vi "IO檔 Enum name 轉換_20200804.vi"() -> ()   [LabVIEW 2019]
uses:
  <vilib>/Utility/file.llb/Read Delimited Spreadsheet (string).vi
panel:
  out "subarray 2":string[](array[string])
  out "subarray":string[](array[string])
  in  "file path (dialog if empty)":path=path "D:/cubtestcsv.csv"
  out "all rows":string[][](array[string])
  out "Array 2":string[](array[string])
  out "Array":string[](array[string])
  in  "Enum":T1(ring)
  in  "Ring":T2 items=["S1-檢平確認氣缸 (設定值)", "$S1_PreventionChk 1", "S1 電路板檢平On次數(設定值)", "$S1_PreventionChk 2", "S1 電池檢平On次數(設定值)", "$S1_PreventionChk 3", "S1 盒蓋檢平On次數(設定值)", "$S1_PreventionChk 4", "S2電流量測 探針使用次數(設定值)", "$S2_PreventionChk 1", "S2-電流量測氣缸 (設定值)", "$S2_PreventionChk 2", "S3程式燒入 探針使用次數(設定值)", "$S3_PreventionChk 1", "S3-程式燒入氣缸 (設定值)", "$S3_PreventionChk 2", "S4電壓量測探針使用次數(設定值)", "$S4_PreventionChk 1", "S4電源3V探針使用次數(設定值)", "$S4_PreventionChk 2", "S4 隔離箱上蓋氣缸 (設定值)", "$S4_PreventionChk 3", "S4 隔離箱下蓋氣缸 (設定值)", "$S4_PreventionChk 4", "S4 電池電壓量測固定氣缸 (設定值)", "$S4_PreventionChk 5", "S4 電池電壓量測氣缸 (設定值)", "$S4_PreventionChk 6", "S4 電路板檢測氣缸(設定值)", "$S4_PreventionChk 7", "S5 電路板取料升降氣缸 (設定值)", "$S5_PreventionChk 1", "S5 電路板取料橫移氣缸 (設定值)", "$S5_PreventionChk 2", "S5 真空 吸取(設定值)", "$S5_PreventionChk 3", "S5 真空 解除(設定值)", "$S5_PreventionChk 4", "S7 焊接料件固定氣缸 (設定值)", "$S7_PreventionChk 1", "S7 焊接機清錫馬達 (設定值)", "$S7_PreventionChk 2", "S10 料件翻轉區升降氣缸 (設定值)", "$S10_PreventionChk 1", "S10 料件翻轉區伸出氣缸 (設定值)", "$S10_PreventionChk 2", "S10 料件翻轉區旋轉氣缸 (設定值)", "$S10_PreventionChk 3", "S10 料件翻轉區夾取氣缸 (設定值)", "$S10_PreventionChk 4", "S10 料件橫移氣缸 (設定值)", "$S10_PreventionChk 5", "S10 料件吸取升降氣缸 (設定值)", "$S10_PreventionChk 6", "S10 料件放料升降氣缸 (設定值)", "$S10_PreventionChk 7", "S10 真空 吸取(設定值)", "$S10_PreventionChk 8", "S10 真空 解除(設定值)", "$S10_PreventionChk 9", "S11 雷射測高檢知氣缸 (設定值)", "$S11_PreventionChk 1", "S12 熱熔升降氣缸 (設定值)", "$S12_PreventionChk 1", "S12 預熱升降氣缸 (設定值)", "$S12_PreventionChk 2", "S12 離子槍風速調控 (設定值)", "$S12_PreventionChk 3", "S13 真空 吸取 (設定值)", "$S13_PreventionChk 1", "S13 真空 解除(設定值)", "$S13_PreventionChk 2", "S13 NG蓋取料夾爪 (設定值)", "$S13_PreventionChk 3", "S13 NG蓋取料升降 (設定值)", "$S13_PreventionChk 4", "S13 NG電池取料升降 (設定值)", "$S13_PreventionChk 5", "S13 NG電路板取料升降 (設定值)", "$S13_PreventionChk 6", "S13 NG橫移氣缸 (設定值)", "$S13_PreventionChk 7", "S13 NG橫移氣缸(設定值)", "$S13_PreventionChk 8", "S7 焊接啟動次數(設定值)", "$S7_PreventionChk 1", "S12 熱熔次數(設定值)", "$S12_PreventionChk 1", "S11 雷射檢測次數(設定值)", "$S11_PreventionChk 1"]
  in  "DIO":cluster{"DI=1":i32, "Name":string[]}[](array[cluster])
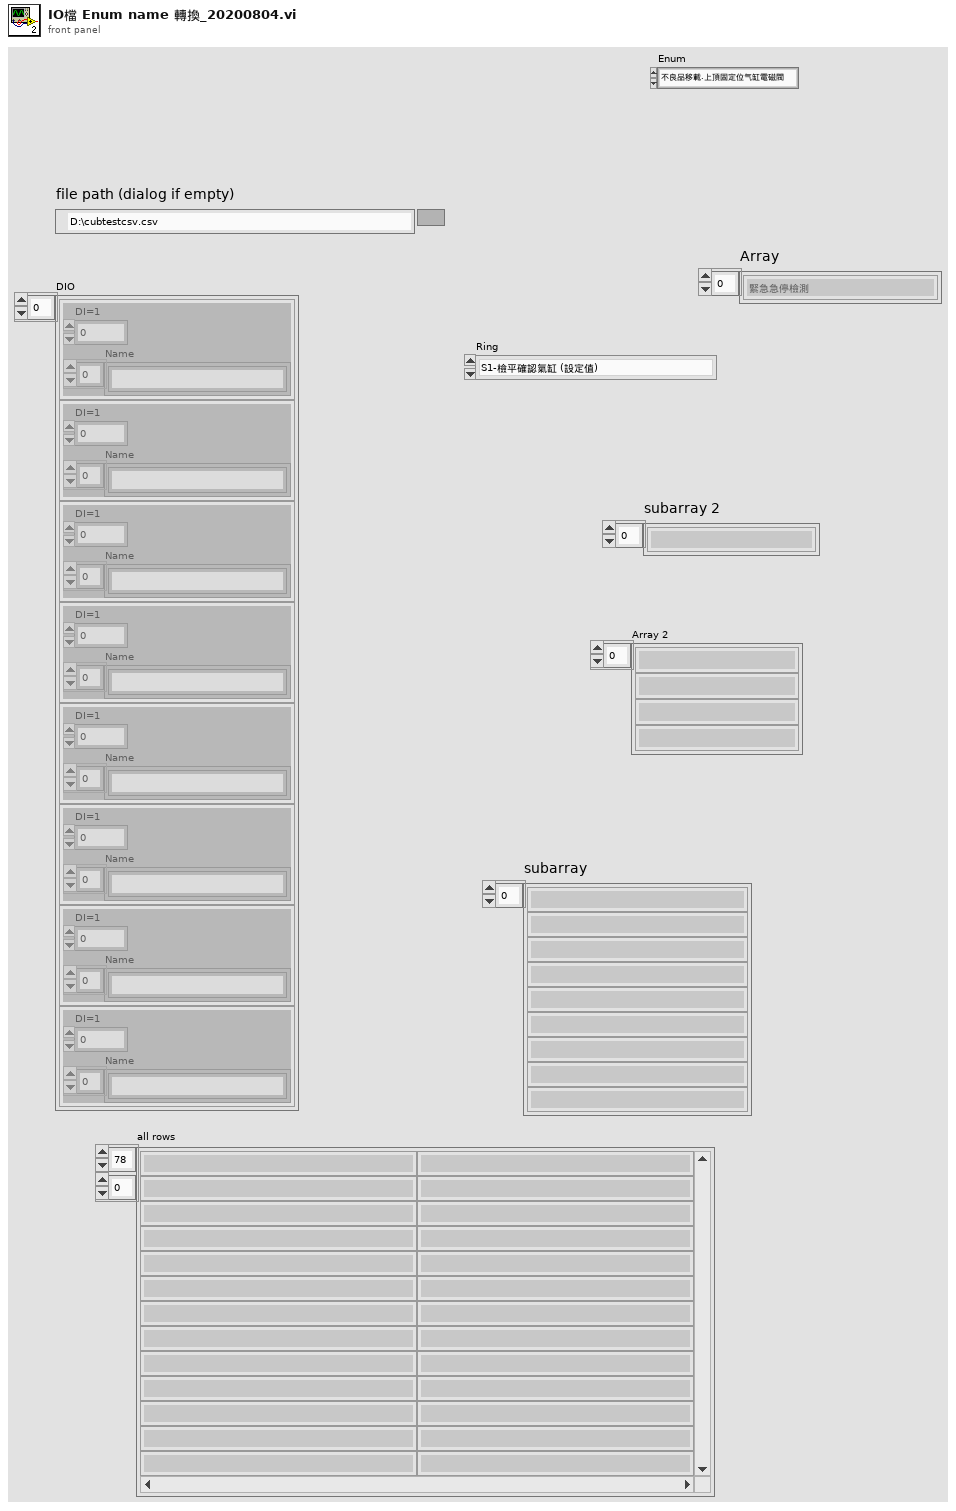
[diagram p1: front panel]
types:
  T1 = enum16{"不良品移載.上頂固定位气缸電磁閥", "不良品移載出料.下壓1氣缸電磁閥", "不良品移載進料.下壓2氣缸電磁閥", "不良品移載.推出料氣缸電磁閥", "不良品移載.推進料氣缸電磁閥"}
  T2 = typedef "預防保養02.ctl" = u16
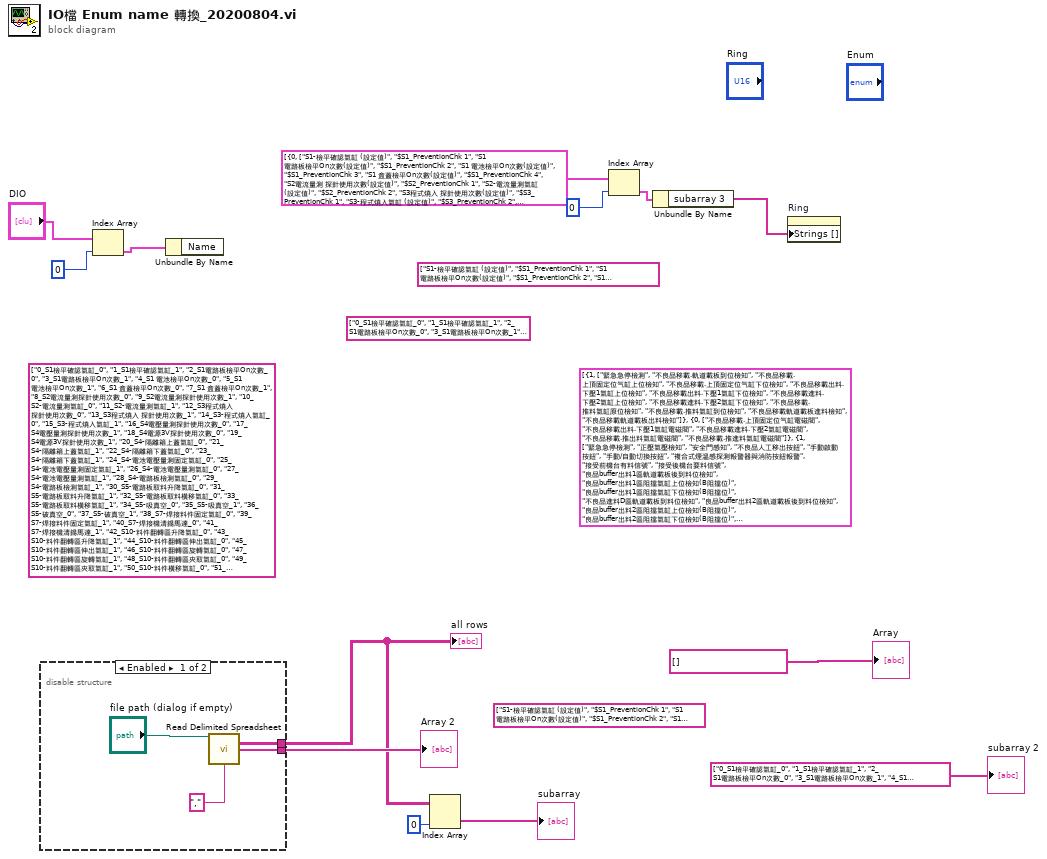
[diagram p0: block diagram]
diagram:
  (unwired) string[] ["S1-檢平確認氣缸 (設定值)", "$S1_PreventionChk 1", "S1 電路板檢平On次數(設定值)", "$S1_PreventionChk 2", "S1 電池檢平On次數(設定值)", "$S1_PreventionChk 3", "S1 盒蓋檢平On次數(設定值)", "$S1_PreventionChk 4", "S2電流量測 探針使用次數(設定值)", "$S2_PreventionChk 1", "S2-電流量測氣缸 (設定值)", "$S2_PreventionChk 2", "S3程式燒入 探針使用次數(設定值)", "$S3_PreventionChk 1", "S3-程式燒入氣缸 (設定值)", "$S3_PreventionChk 2", "S4電壓量測探針使用次數(設定值)", "$S4_PreventionChk 1", "S4電源3V探針使用次數(設定值)", "$S4_PreventionChk 2", "S4 隔離箱上蓋氣缸 (設定值)", "$S4_PreventionChk 3", "S4 隔離箱下蓋氣缸 (設定值)", "$S4_PreventionChk 4", "S4 電池電壓量測固定氣缸 (設定值)", "$S4_PreventionChk 5", "S4 電池電壓量測氣缸 (設定值)", "$S4_PreventionChk 6", "S4 電路板檢測氣缸(設定值)", "$S4_PreventionChk 7", "S5 電路板取料升降氣缸 (設定值)", "$S5_PreventionChk 1", "S5 電路板取料橫移氣缸 (設定值)", "$S5_PreventionChk 2", "S5 真空 吸取(設定值)", "$S5_PreventionChk 3", "S5 真空 解除(設定值)", "$S5_PreventionChk 4", "S7 焊接料件固定氣缸 (設定值)", "$S7_PreventionChk 1", "S7 焊接機清錫馬達 (設定值)", "$S7_PreventionChk 2", "S10 料件翻轉區升降氣缸 (設定值)", "$S10_PreventionChk 1", "S10 料件翻轉區伸出氣缸 (設定值)", "$S10_PreventionChk 2", "S10 料件翻轉區旋轉氣缸 (設定值)", "$S10_PreventionChk 3", "S10 料件翻轉區夾取氣缸 (設定值)", "$S10_PreventionChk 4", "S10 料件橫移氣缸 (設定值)", "$S10_PreventionChk 5", "S10 料件吸取升降氣缸 (設定值)", "$S10_PreventionChk 6", "S10 料件放料升降氣缸 (設定值)", "$S10_PreventionChk 7", "S10 真空 吸取(設定值)", "$S10_PreventionChk 8", "S10 真空 解除(設定值)", "$S10_PreventionChk 9", "S11 雷射測高檢知氣缸 (設定值)", "$S11_PreventionChk 1", "S12 熱熔升降氣缸 (設定值)", "$S12_PreventionChk 1", "S12 預熱升降氣缸 (設定值)", "$S12_PreventionChk 2", "S12 離子槍風速調控 (設定值)", "$S12_PreventionChk 3", "S13 真空 吸取 (設定值)", "$S13_PreventionChk 1", "S13 真空 解除(設定值)", "$S13_PreventionChk 2", "S13 NG蓋取料夾爪 (設定值)", "$S13_PreventionChk 3", "S13 NG蓋取料升降 (設定值)", "$S13_PreventionChk 4", "S13 NG電池取料升降 (設定值)", "$S13_PreventionChk 5", "S13 NG電路板取料升降 (設定值)", "$S13_PreventionChk 6", "S13 NG橫移氣缸 (設定值)", "$S13_PreventionChk 7", "S13 NG橫移氣缸(設定值)", "$S13_PreventionChk 8", "S7 焊接啟動次數(設定值)", "$S7_PreventionChk 1", "S12 熱熔次數(設定值)", "$S12_PreventionChk 4", "S11 雷射檢測次數(設定值)", "$S11_PreventionChk 1"] ("subarray 3")
  (unwired) string[] ["S1-檢平確認氣缸 (設定值)", "$S1_PreventionChk 1", "S1 電路板檢平On次數(設定值)", "$S1_PreventionChk 2", "S1 電池檢平On次數(設定值)", "$S1_PreventionChk 3", "S1 盒蓋檢平On次數(設定值)", "$S1_PreventionChk 4", "S2電流量測 探針使用次數(設定值)", "$S2_PreventionChk 1", "S2-電流量測氣缸 (設定值)", "$S2_PreventionChk 2", "S3程式燒入 探針使用次數(設定值)", "$S3_PreventionChk 1", "S3-程式燒入氣缸 (設定值)", "$S3_PreventionChk 2", "S4電壓量測探針使用次數(設定值)", "$S4_PreventionChk 1", "S4電源3V探針使用次數(設定值)", "$S4_PreventionChk 2", "S4 隔離箱上蓋氣缸 (設定值)", "$S4_PreventionChk 3", "S4 隔離箱下蓋氣缸 (設定值)", "$S4_PreventionChk 4", "S4 電池電壓量測固定氣缸 (設定值)", "$S4_PreventionChk 5", "S4 電池電壓量測氣缸 (設定值)", "$S4_PreventionChk 6", "S4 電路板檢測氣缸(設定值)", "$S4_PreventionChk 7", "S5 電路板取料升降氣缸 (設定值)", "$S5_PreventionChk 1", "S5 電路板取料橫移氣缸 (設定值)", "$S5_PreventionChk 2", "S5 真空 吸取(設定值)", "$S5_PreventionChk 3", "S5 真空 解除(設定值)", "$S5_PreventionChk 4", "S7 焊接料件固定氣缸 (設定值)", "$S7_PreventionChk 1", "S7 焊接機清錫馬達 (設定值)", "$S7_PreventionChk 2", "S10 料件翻轉區升降氣缸 (設定值)", "$S10_PreventionChk 1", "S10 料件翻轉區伸出氣缸 (設定值)", "$S10_PreventionChk 2", "S10 料件翻轉區旋轉氣缸 (設定值)", "$S10_PreventionChk 3", "S10 料件翻轉區夾取氣缸 (設定值)", "$S10_PreventionChk 4", "S10 料件橫移氣缸 (設定值)", "$S10_PreventionChk 5", "S10 料件吸取升降氣缸 (設定值)", "$S10_PreventionChk 6", "S10 料件放料升降氣缸 (設定值)", "$S10_PreventionChk 7", "S10 真空 吸取(設定值)", "$S10_PreventionChk 8", "S10 真空 解除(設定值)", "$S10_PreventionChk 9", "S11 雷射測高檢知氣缸 (設定值)", "$S11_PreventionChk 1", "S12 熱熔升降氣缸 (設定值)", "$S12_PreventionChk 1", "S12 預熱升降氣缸 (設定值)", "$S12_PreventionChk 2", "S12 離子槍風速調控 (設定值)", "$S12_PreventionChk 3", "S13 真空 吸取 (設定值)", "$S13_PreventionChk 1", "S13 真空 解除(設定值)", "$S13_PreventionChk 2", "S13 NG蓋取料夾爪 (設定值)", "$S13_PreventionChk 3", "S13 NG蓋取料升降 (設定值)", "$S13_PreventionChk 4", "S13 NG電池取料升降 (設定值)", "$S13_PreventionChk 5", "S13 NG電路板取料升降 (設定值)", "$S13_PreventionChk 6", "S13 NG橫移氣缸 (設定值)", "$S13_PreventionChk 7", "S13 NG橫移氣缸(設定值)", "$S13_PreventionChk 8", "S7 焊接啟動次數(設定值)", "$S7_PreventionChk 1", "S12 熱熔次數(設定值)", "$S12_PreventionChk 1", "S11 雷射檢測次數(設定值)", "$S11_PreventionChk 1"] ("subarray 3")
  (unwired) string[] ["0_S1檢平確認氣缸_0", "1_S1檢平確認氣缸_1", "2_S1電路板檢平On次數_0", "3_S1電路板檢平On次數_1", "4_S1 電池檢平On次數_0", "5_S1 電池檢平On次數_1", "6_S1 盒蓋檢平On次數_0", "7_S1 盒蓋檢平On次數_1", "8_S2電流量測探針使用次數_0", "9_S2電流量測探針使用次數_1", "10_S2-電流量測氣缸_0", "11_S2-電流量測氣缸_1", "12_S3程式燒入 探針使用次數_0", "13_S3程式燒入 探針使用次數_1", "14_S3-程式燒入氣缸_0", "15_S3-程式燒入氣缸_1", "16_S4電壓量測探針使用次數_0", "17_S4電壓量測探針使用次數_1", "18_S4電源3V探針使用次數_0", "19_S4電源3V探針使用次數_1", "20_S4-隔離箱上蓋氣缸_0", "21_S4-隔離箱上蓋氣缸_1", "22_S4-隔離箱下蓋氣缸_0", "23_S4-隔離箱下蓋氣缸_1", "24_S4-電池電壓量測固定氣缸_0", "25_S4-電池電壓量測固定氣缸_1", "26_S4-電池電壓量測氣缸_0", "27_S4-電池電壓量測氣缸_1", "28_S4-電路板檢測氣缸_0", "29_S4-電路板檢測氣缸_1", "30_S5-電路板取料升降氣缸_0", "31_S5-電路板取料升降氣缸_1", "32_S5-電路板取料橫移氣缸_0", "33_S5-電路板取料橫移氣缸_1", "34_S5-吸真空_0", "35_S5-吸真空_1", "36_S5-破真空_0", "37_S5-破真空_1", "38_S7-焊接料件固定氣缸_0", "39_S7-焊接料件固定氣缸_1", "40_S7-焊接機清錫馬達_0", "41_S7-焊接機清錫馬達_1", "42_S10-料件翻轉區升降氣缸_0", "43_S10-料件翻轉區升降氣缸_1", "44_S10-料件翻轉區伸出氣缸_0", "45_S10-料件翻轉區伸出氣缸_1", "46_S10-料件翻轉區旋轉氣缸_0", "47_S10-料件翻轉區旋轉氣缸_1", "48_S10-料件翻轉區夾取氣缸_0", "49_S10-料件翻轉區夾取氣缸_1", "50_S10-料件橫移氣缸_0", "51_S10-料件橫移氣缸_1", "52_S10-料件吸取升降氣缸_0", "53_S10-料件吸取升降氣缸_1", "54_S10-料件放料升降氣缸_0", "55_S10-料件放料升降氣缸_1", "56_S10-吸真空_0", "57_S10-吸真空_1", "58_S10-破真空_0", "59_S10-破真空_1", "60_S11-雷射測高檢知氣缸_0", "61_S11-雷射測高檢知氣缸_1", "62_S12-熱熔升降氣缸_0", "63_S12-熱熔升降氣缸_1", "64_S12-預熱升降氣缸_0", "65_S12-預熱升降氣缸_1", "66_S12-離子槍風速調控_0", "67_S12-離子槍風速調控_1", "68_S13-吸真空_0", "69_S13-吸真空_1", "70_S13-破真空_0", "71_S13-破真空_1", "72_S13-NG蓋取料夾爪_0", "73_S13-NG蓋取料夾爪_1", "74_S13-NG蓋取料升降_0", "75_S13-NG蓋取料升降_1", "76_S13-NG電池取料升降_0", "77_S13-NG電池取料升降_1", "78_S13-NG電路板取料升降_0", "79_S13-NG電路板取料升降_1", "80_S13-NG橫移氣缸_0", "81_S13-NG橫移氣缸_1", "82_S13-NG橫移氣缸_0", "83_S13-NG橫移氣缸_1", "84_S7-焊接啟動次數_0", "85_S7-焊接啟動次數_1", "86_S12-熱熔次數_0", "87_S12-熱熔次數_1", "88_S11-雷射檢測次數_0", "89_S11-雷射檢測次數_1"] ("subarray 2")
  (unwired) string[] ["0_S1檢平確認氣缸_0", "1_S1檢平確認氣缸_1", "2_S1電路板檢平On次數_0", "3_S1電路板檢平On次數_1", "4_S1 電池檢平On次數_0", "5_S1 電池檢平On次數_1", "6_S1 盒蓋檢平On次數_0", "7_S1 盒蓋檢平On次數_1", "8_S2電流量測探針使用次數_0", "9_S2電流量測探針使用次數_1", "10_S2-電流量測氣缸_0", "11_S2-電流量測氣缸_1", "12_S3程式燒入 探針使用次數_0", "13_S3程式燒入 探針使用次數_1", "14_S3-程式燒入氣缸_0", "15_S3-程式燒入氣缸_1", "16_S4電壓量測探針使用次數_0", "17_S4電壓量測探針使用次數_1", "18_S4電源3V探針使用次數_0", "19_S4電源3V探針使用次數_1", "20_S4-隔離箱上蓋氣缸_0", "21_S4-隔離箱上蓋氣缸_1", "22_S4-隔離箱下蓋氣缸_0", "23_S4-隔離箱下蓋氣缸_1", "24_S4-電池電壓量測固定氣缸_0", "25_S4-電池電壓量測固定氣缸_1", "26_S4-電池電壓量測氣缸_0", "27_S4-電池電壓量測氣缸_1", "28_S4-電路板檢測氣缸_0", "29_S4-電路板檢測氣缸_1", "30_S5-電路板取料升降氣缸_0", "31_S5-電路板取料升降氣缸_1", "32_S5-電路板取料橫移氣缸_0", "33_S5-電路板取料橫移氣缸_1", "34_S5-吸真空_0", "35_S5-吸真空_1", "36_S5-破真空_0", "37_S5-破真空_1", "38_S7-焊接料件固定氣缸_0", "39_S7-焊接料件固定氣缸_1", "40_S7-焊接機清錫馬達_0", "41_S7-焊接機清錫馬達_1", "42_S10-料件翻轉區升降氣缸_0", "43_S10-料件翻轉區升降氣缸_1", "44_S10-料件翻轉區伸出氣缸_0", "45_S10-料件翻轉區伸出氣缸_1", "46_S10-料件翻轉區旋轉氣缸_0", "47_S10-料件翻轉區旋轉氣缸_1", "48_S10-料件翻轉區夾取氣缸_0", "49_S10-料件翻轉區夾取氣缸_1", "50_S10-料件橫移氣缸_0", "51_S10-料件橫移氣缸_1", "52_S10-料件吸取升降氣缸_0", "53_S10-料件吸取升降氣缸_1", "54_S10-料件放料升降氣缸_0", "55_S10-料件放料升降氣缸_1", "56_S10-吸真空_0", "57_S10-吸真空_1", "58_S10-破真空_0", "59_S10-破真空_1", "60_S11-雷射測高檢知氣缸_0", "61_S11-雷射測高檢知氣缸_1", "62_S12-熱熔升降氣缸_0", "63_S12-熱熔升降氣缸_1", "64_S12-預熱升降氣缸_0", "65_S12-預熱升降氣缸_1", "66_S12-離子槍風速調控_0", "67_S12-離子槍風速調控_1", "68_S13-吸真空_0", "69_S13-吸真空_1", "70_S13-破真空_0", "71_S13-破真空_1", "72_S13-NG蓋取料夾爪_0", "73_S13-NG蓋取料夾爪_1", "74_S13-NG蓋取料升降_0", "75_S13-NG蓋取料升降_1", "76_S13-NG電池取料升降_0", "77_S13-NG電池取料升降_1", "78_S13-NG電路板取料升降_0", "79_S13-NG電路板取料升降_1", "80_S13-NG橫移氣缸_0", "81_S13-NG橫移氣缸_1", "82_S13-NG橫移氣缸_0", "83_S13-NG橫移氣缸_1", "84_S7-焊接啟動次數_0", "85_S7-焊接啟動次數_1", "86_S12-熱熔次數_0", "87_S12-熱熔次數_1", "88_S11-雷射檢測次數_0", "89_S11-雷射檢測次數_1"] ("subarray 2")
  (unwired) cluster{"DI=1":i32, "Name":string[]}[] [{"DI=1"=1, "Name"=["緊急急停檢測", "不良品移載.軌道載板到位檢知", "不良品移載.上頂固定位气缸上位檢知", "不良品移載.上頂固定位气缸下位檢知", "不良品移載出料.下壓1氣缸上位檢知", "不良品移載出料.下壓1氣缸下位檢知", "不良品移載進料.下壓2氣缸上位檢知", "不良品移載進料.下壓2氣缸下位檢知", "不良品移載.推料氣缸原位檢知", "不良品移載.推料氣缸到位檢知", "不良品移載軌道載板進料檢知", "不良品移載軌道載板出料檢知"]}, {"DI=1"=0, "Name"=["不良品移載.上頂固定位气缸電磁閥", "不良品移載出料.下壓1氣缸電磁閥", "不良品移載進料.下壓2氣缸電磁閥", "不良品移載.推出料氣缸電磁閥", "不良品移載.推進料氣缸電磁閥"]}, {"DI=1"=1, "Name"=["緊急急停檢測", "正壓氣壓檢知", "安全門感知", "不良品人工移出按鈕", "手動啟動 按鈕", "手動/自動切換按鈕", "複合式煙溫感探測報警器與消防按鈕報警", "接受前機台有料信號", "接受後機台要料信號", "良品buffer出料1區軌道載板後到料位檢知", "良品buffer出料1區阻擋氣缸上位檢知(B阻擋位)", "良品buffer出料1區阻擋氣缸下位檢知(B阻擋位)", "不良品進料D區軌道載板到料位檢知", "良品buffer出料2區軌道載板後到料位檢知", "良品buffer出料2區阻擋氣缸上位檢知(B阻擋位)", "良品buffer出料2區阻擋氣缸下位檢知(B阻擋位)", "不良品進料C區軌道載板到料位檢知", "良品buffer出料3區軌道載板後到料位檢知", "良品buffer出料3區阻擋氣缸上位檢知(B阻擋位)", "良品buffer出料3區阻擋氣缸下位檢知(B阻擋位)", "不良品進料B區軌道載板後到料位檢知", "良品buffer出料4區軌道載板到料位檢知", "良品buffer出料4區阻擋氣缸上位檢知(B阻擋位)", "良品buffer出料4區阻擋氣缸下位檢知(B阻擋位)", "不良品進料A區軌道載板到料位檢知", "不良品出料5區軌道載板後到料位檢知", "不良品出料5區阻擋氣缸上位檢知(A阻擋位)", "不良品出料5區阻擋氣缸下位檢知(A阻擋位)", "手動良品進料按鈕"]}, {"DI=1"=0, "Name"=["蜂鳴器", "紅燈", "綠燈", "黃燈", "向前機發出要料信號", "通知後機站有料輸出信號", "不良品buffer區馬達啟動", "不良品buffer區馬達正轉/反轉", "良品buffer出料1區阻擋氣缸電磁閥", "良品buffer出料2區阻擋氣缸電磁閥", "良品buffer出料3區阻擋氣缸電磁閥", "良品buffer出料4區阻擋氣缸電磁閥", "不良品出料5區阻擋氣缸電磁閥"]}] ("DIO")
  n1 = disable-structure shown="Enabled" {
    disable-tunnel: [w16 _] -> w5
    disable-tunnel: [w15 _] -> w4
    frame Enabled {
      n2 = call-poly <vilib>:"Read Delimited Spreadsheet.vi"("file path (dialog if empty)"="file path (dialog if empty)", "delimiter (\\t)"="," ("delimiter (\\t)")) -> ("all rows"=w15:string[][], "first row"=w16:string[])  [unwired: 8 in, 4 out]
    }
    frame Disabled {
    }
  }
  "Array 2" <- w5
  "all rows" <- w4
  n3 = Index Array(array="DIO", index=0) -> (element=w11:cluster{"DI=1":i32, "Name":string[]})
  n4 = Unbundle By Name(w11) -> ()  [unwired: 1 out]
  n5 = Index Array(array=w4, index (col)=0 ("disabled index (col)")) -> (element=→"subarray":string[])  [unwired: 1 in]
  n6 = Index Array(array=cluster{"DI=1":i32, "subarray 3":string[]}[] [{"DI=1"=0, "subarray 3"=["S1-檢平確認氣缸 (設定值)", "$S1_PreventionChk 1", "S1 電路板檢平On次數(設定值)", "$S1_PreventionChk 2", "S1 電池檢平On次數(設定值)", "$S1_PreventionChk 3", "S1 盒蓋檢平On次數(設定值)", "$S1_PreventionChk 4", "S2電流量測 探針使用次數(設定值)", "$S2_PreventionChk 1", "S2-電流量測氣缸 (設定值)", "$S2_PreventionChk 2", "S3程式燒入 探針使用次數(設定值)", "$S3_PreventionChk 1", "S3-程式燒入氣缸 (設定值)", "$S3_PreventionChk 2", "S4電壓量測探針使用次數(設定值)", "$S4_PreventionChk 1", "S4電源3V探針使用次數(設定值)", "$S4_PreventionChk 2", "S4 隔離箱上蓋氣缸 (設定值)", "$S4_PreventionChk 3", "S4 隔離箱下蓋氣缸 (設定值)", "$S4_PreventionChk 4", "S4 電池電壓量測固定氣缸 (設定值)", "$S4_PreventionChk 5", "S4 電池電壓量測氣缸 (設定值)", "$S4_PreventionChk 6", "S4 電路板檢測氣缸(設定值)", "$S4_PreventionChk 7", "S5 電路板取料升降氣缸 (設定值)", "$S5_PreventionChk 1", "S5 電路板取料橫移氣缸 (設定值)", "$S5_PreventionChk 2", "S5 真空 吸取(設定值)", "$S5_PreventionChk 3", "S5 真空 解除(設定值)", "$S5_PreventionChk 4", "S7 焊接料件固定氣缸 (設定值)", "$S7_PreventionChk 1", "S7 焊接機清錫馬達 (設定值)", "$S7_PreventionChk 2", "S10 料件翻轉區升降氣缸 (設定值)", "$S10_PreventionChk 1", "S10 料件翻轉區伸出氣缸 (設定值)", "$S10_PreventionChk 2", "S10 料件翻轉區旋轉氣缸 (設定值)", "$S10_PreventionChk 3", "S10 料件翻轉區夾取氣缸 (設定值)", "$S10_PreventionChk 4", "S10 料件橫移氣缸 (設定值)", "$S10_PreventionChk 5", "S10 料件吸取升降氣缸 (設定值)", "$S10_PreventionChk 6", "S10 料件放料升降氣缸 (設定值)", "$S10_PreventionChk 7", "S10 真空 吸取(設定值)", "$S10_PreventionChk 8", "S10 真空 解除(設定值)", "$S10_PreventionChk 9", "S11 雷射測高檢知氣缸 (設定值)", "$S11_PreventionChk 1", "S12 熱熔升降氣缸 (設定值)", "$S12_PreventionChk 1", "S12 預熱升降氣缸 (設定值)", "$S12_PreventionChk 2", "S12 離子槍風速調控 (設定值)", "$S12_PreventionChk 3", "S13 真空 吸取 (設定值)", "$S13_PreventionChk 1", "S13 真空 解除(設定值)", "$S13_PreventionChk 2", "S13 NG蓋取料夾爪 (設定值)", "$S13_PreventionChk 3", "S13 NG蓋取料升降 (設定值)", "$S13_PreventionChk 4", "S13 NG電池取料升降 (設定值)", "$S13_PreventionChk 5", "S13 NG電路板取料升降 (設定值)", "$S13_PreventionChk 6", "S13 NG橫移氣缸 (設定值)", "$S13_PreventionChk 7", "S13 NG橫移氣缸(設定值)", "$S13_PreventionChk 8", "S7 焊接啟動次數(設定值)", "$S7_PreventionChk 1", "S12 熱熔次數(設定值)", "$S12_PreventionChk 1", "S11 雷射檢測次數(設定值)", "$S11_PreventionChk 1"]}] ("DIO"), index=0) -> (element=w9:cluster{"DI=1":i32, "subarray 3":string[]})
  n7 = Unbundle By Name(w9) -> ("subarray 3"=w8:string[])
  n8 = property on="Ring" class="Ring (strict)"("Strings []"=w8) -> ()  [unwired: 2 in, 2 out]
  "Array" <- string[] []
  "subarray 2" <- string[] ["0_S1檢平確認氣缸_0", "1_S1檢平確認氣缸_1", "2_S1電路板檢平On次數_0", "3_S1電路板檢平On次數_1", "4_S1 電池檢平On次數_0", "5_S1 電池檢平On次數_1", "6_S1 盒蓋檢平On次數_0", "7_S1 盒蓋檢平On次數_1", "8_S2電流量測探針使用次數_0", "9_S2電流量測探針使用次數_1", "10_S2-電流量測氣缸_0", "11_S2-電流量測氣缸_1", "12_S3程式燒入 探針使用次數_0", "13_S3程式燒入 探針使用次數_1", "14_S3-程式燒入氣缸_0", "15_S3-程式燒入氣缸_1", "16_S4電壓量測探針使用次數_0", "17_S4電壓量測探針使用次數_1", "18_S4電源3V探針使用次數_0", "19_S4電源3V探針使用次數_1", "20_S4-隔離箱上蓋氣缸_0", "21_S4-隔離箱上蓋氣缸_1", "22_S4-隔離箱下蓋氣缸_0", "23_S4-隔離箱下蓋氣缸_1", "24_S4-電池電壓量測固定氣缸_0", "25_S4-電池電壓量測固定氣缸_1", "26_S4-電池電壓量測氣缸_0", "27_S4-電池電壓量測氣缸_1", "28_S4-電路板檢測氣缸_0", "29_S4-電路板檢測氣缸_1", "30_S5-電路板取料升降氣缸_0", "31_S5-電路板取料升降氣缸_1", "32_S5-電路板取料橫移氣缸_0", "33_S5-電路板取料橫移氣缸_1", "34_S5-吸真空_0", "35_S5-吸真空_1", "36_S5-破真空_0", "37_S5-破真空_1", "38_S7-焊接料件固定氣缸_0", "39_S7-焊接料件固定氣缸_1", "40_S7-焊接機清錫馬達_0", "41_S7-焊接機清錫馬達_1", "42_S10-料件翻轉區升降氣缸_0", "43_S10-料件翻轉區升降氣缸_1", "44_S10-料件翻轉區伸出氣缸_0", "45_S10-料件翻轉區伸出氣缸_1", "46_S10-料件翻轉區旋轉氣缸_0", "47_S10-料件翻轉區旋轉氣缸_1", "48_S10-料件翻轉區夾取氣缸_0", "49_S10-料件翻轉區夾取氣缸_1", "50_S10-料件橫移氣缸_0", "51_S10-料件橫移氣缸_1", "52_S10-料件吸取升降氣缸_0", "53_S10-料件吸取升降氣缸_1", "54_S10-料件放料升降氣缸_0", "55_S10-料件放料升降氣缸_1", "56_S10-吸真空_0", "57_S10-吸真空_1", "58_S10-破真空_0", "59_S10-破真空_1", "60_S11-雷射測高檢知氣缸_0", "61_S11-雷射測高檢知氣缸_1", "62_S12-熱熔升降氣缸_0", "63_S12-熱熔升降氣缸_1", "64_S12-預熱升降氣缸_0", "65_S12-預熱升降氣缸_1", "66_S12-離子槍風速調控_0", "67_S12-離子槍風速調控_1", "68_S13-吸真空_0", "69_S13-吸真空_1", "70_S13-破真空_0", "71_S13-破真空_1", "72_S13-NG蓋取料夾爪_0", "73_S13-NG蓋取料夾爪_1", "74_S13-NG蓋取料升降_0", "75_S13-NG蓋取料升降_1", "76_S13-NG電池取料升降_0", "77_S13-NG電池取料升降_1", "78_S13-NG電路板取料升降_0", "79_S13-NG電路板取料升降_1", "80_S13-NG橫移氣缸_0", "81_S13-NG橫移氣缸_1", "82_S13-NG橫移氣缸_0", "83_S13-NG橫移氣缸_1", "84_S7-焊接啟動次數_0", "85_S7-焊接啟動次數_1", "86_S12-熱熔次數_0", "87_S12-熱熔次數_1", "88_S11-雷射檢測次數_0", "89_S11-雷射檢測次數_1"] ("subarray 2")
